vi "Set 3DM-GX3-45.vi"   [LabVIEW 2012]
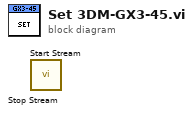
[diagram p0: block diagram]
diagram:
  n1 = call "Stop Stream.vi"() -> ()  [unwired: 10 in, 2 out]
  n2 = call "Start Stream.vi"() -> ()  [unwired: 10 in, 2 out]
